vi "Handle Error.vi"(8 "error in (no error)":errorcluster, 11 "TestLNA in":refnum<class "TestLNA.lvclass">) -> (0 "error out":errorcluster, 2 "stop actor?":bool=TRUE, 3 "TestLNA out":refnum<class "TestLNA.lvclass">)   [LabVIEW 2014, in "TestLNA.lvlib" / "TestLNA.lvclass"]
doc: "(<B>Filename</B>: Actor Framework.lvlib:Actor.lvclass:Handle Error.vi)\n\nDefines how the actor handles an error that occurred while processing a message.\n\nBy default, this method does nothing except stop the actor. This method also treats error code 43 (coming from <B>error in</B>) as a sign that the actor shut down normally. In this situation, the Handle Error method does not return the error on <B>error out</B>, meaning the actor's caller will not receive it. All other error codes will be returned on <B>error out</B>.\n\nA descendant class may override this method to change this behavior."
uses:
  TestLNA.lvclass
  CSPP_LNA/CS++LNAMessage.lvclass
  CSPP_LNA/CS++LNAMessage.lvclass/CS++LNAMessage.ctl
  TestLNA.lvclass/TestLNA.ctl
  LNA Messages/LNA Return Message Msg/LNA Return Message Msg.lvclass
  <vilib>/NI/Actors/Linked Network Actor/Linked Network Actor Messages/LNA Return Message Msg/LNA Return Message Msg.lvclass/LNA Return Message Msg.ctl
  <vilib>/ActorFramework/Actor/Actor.lvclass/Actor.ctl
  <vilib>/ActorFramework/Message Enqueuer/Message Enqueuer.lvclass/Message Enqueuer.ctl
  CSPP_LNA/Write Message Class Name.vi
  CSPP_LNA/Write Parameter.vi
  <vilib>/ActorFramework/Message Enqueuer/Init from Existing Queue.vi
  <vilib>/ActorFramework/Message Priority Queue/Priority Enqueue.vi
  <vilib>/ActorFramework/Message Enqueuer/Message Enqueuer.lvclass
  CSPP_Core/Actors/CS++BaseActor/CS++BaseActor.lvclass
  <vilib>/NI/Actors/Linked Network Actor/Linked Network Actor Messages/Transmit Network Message Msg/Transmit Network Message Msg.lvclass
  <vilib>/NI/Actors/Linked Network Actor/Linked Network Actor Messages/LNA Return Message Msg/LNA Return Message Msg.lvclass
  <vilib>/ActorFramework/Actor/Actor.lvclass
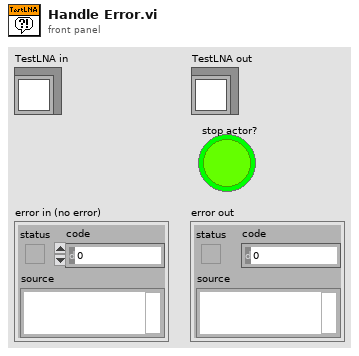
[diagram p1: front panel]
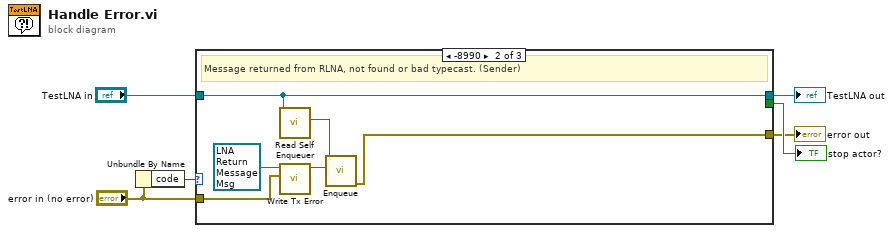
[diagram p0: block diagram]
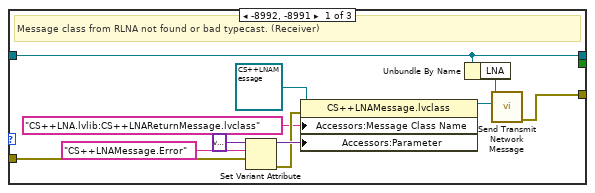
[diagram p2: hidden frame]
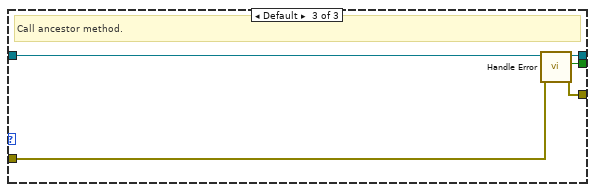
[diagram p3: hidden frame]
diagram:
  n1 = Unbundle By Name("error in (no error)") -> ("code"=w4:i32)
  n2 = case shown="-8990" w4 {
    tunnel: [w17 w18 w26] -> w1
    tunnel: [w15 w21 w25] -> w2
    tunnel: "error in (no error)" -> [w9 w23 w27]
    tunnel: "TestLNA in" -> [w15 w21 w28]
    tunnel: [_ _ w24] -> w3
    frame -8992, -8991 {
      # "Message class from RLNA not found or bad typecast. (Receiver)"
      n3 = Set Variant Attribute(Variant=variant, name="CS++LNAMessage.Error", value=w9) -> (Variant out=w13:variant, error out=w10:errorcluster)  [unwired: 1 in, 1 out]
      n4 = property class="CS++LNAMessage.lvclass"(reference=refnum<class "CS++LNAMessage.lvclass"> refnum ("CS++LNA.lvlib:CS++LNAMessage.lvclass"), error in=w10, "Accessors:Message Class Name"="CS++LNA.lvlib:CS++LNAReturnMessage.lvclass" ("Message Class Name"), "Accessors:Parameter"=w13) -> (reference out=w8:refnum<class "CS++LNAMessage.lvclass">)  [unwired: 1 out]
      n5 = Unbundle By Name(w15) -> ("LNA"=w16:refnum<class "Message Enqueuer.lvclass">)
      n6 = call <vilib>:"Send Transmit Network Message.vi"("Message"=w8, "Message Enqueuer"=w16) -> ("error out"=w17:errorcluster)  [unwired: 8 in, 1 out]
    }
    frame -8990 {
      # "Message returned from RLNA, not found or bad typecast. (Sender)"
      n7 = call <vilib>:"Read Self Enqueuer.vi"("Actor"=w21) -> ("Self Enqueuer"=w20:refnum<class "Message Enqueuer.lvclass">)  [unwired: 10 in]
      n8 = call <vilib>:"Write Tx Error.vi"("Tx Error"=w23, "LNA Return Message Msg in"=refnum<class "LNA Return Message Msg.lvclass"> refnum ("TestLNA.lvlib:LNA Return Message Msg.lvclass")) -> ("LNA Return Message Msg out"=w19:refnum<class "LNA Return Message Msg.lvclass">)  [unwired: 8 in, 1 out]
      n9 = call <vilib>:"Enqueue.vi"("Message"=w19, "Message Enqueuer in"=w20) -> ("error out"=w18:errorcluster)  [unwired: 8 in, 1 out]
    }
    frame Default {
      # "Call ancestor method."
      n10 = call-parent "Handle Error.vi"("error in (no error)"=w27, "CS++BaseActor in"=w28) -> ("error out"=w26:errorcluster, "stop actor?"=w24:bool, "CS++BaseActor out"=w25:refnum<class "TestLNA.lvclass">)  [unwired: 7 in]
    }
  }
  "TestLNA out" <- w2
  "error out" <- w1
  "stop actor?" <- w3
